vi "HFRR ADV v08.vi"() -> ()   [LabVIEW 2025] (continued)
                  }
                  frame True {
                    w544 = 0.0 ("Major Axis")
                    n250 = Match Pattern(string=w549, regular expression="\"length_px\":") -> (after substring=w547:string)  [unwired: 1 in, 3 out]
                    n251 = property on="Major Axis" class="DigNum (strict)"("Caption.Text"="") -> ()  [unwired: 2 in, 2 out]
                    n252 = property on="Minor Axis" class="DigNum (strict)"("Caption.Text"="") -> ()  [unwired: 2 in, 2 out]
                    n253 = property on="Average" class="DigNum (strict)"("Caption.Text"="Line") -> ()  [unwired: 2 in, 2 out]
                    n254 = Fract/Exp String To Number(string=w547, default (0 dbl)=0.0 ("default (0 DBL)")) -> (number=w543:dbl)  [unwired: 2 in, 1 out]
                    "Pixel Value" <- w543
                    n255 = Multiply(x=w543, y=w545) -> (x*y=w556:dbl)
                    n256 = Multiply(x=w556, y=1000.0) -> (x*y=w539:dbl)
                    n257 = Divide(x=w539, y=1000.0) -> (x/y=w542:dbl)
                    n258 = local write "Measurment (mm)"(w542) -> ()
                    n259 = Bundle By Name(cluster=w548, "average"=w539) -> (w546:cluster{"major":dbl, "minor":dbl, "average":dbl})
                    n260 = Number To Fractional String(number=w539, precision (6)=i16 1) -> (F-format string=w538:string)  [unwired: 2 in]
                    n261 = local write "Minor Axis"(w544) -> ()
                    n262 = local write "Major Axis"(w544) -> ()
                    n263 = Fract/Exp String To Number(string=w538) -> (number=w537:dbl)  [unwired: 3 in, 1 out]
                    n264 = local write "Average"(w537) -> ()
                  }
                }
              }
              frame True {
                w576 = 1000.0 ("y")
                w582 = 0.0 ("default (0 DBL)")
                n265 = Match Pattern(string=w588, regular expression=" \"width_px\":") -> (after substring=w586:string)  [unwired: 1 in, 3 out]
                n266 = Match Pattern(string=w586, regular expression="\"height_px\":") -> (before substring=w584:string, after substring=w583:string)  [unwired: 1 in, 2 out]
                n267 = Fract/Exp String To Number(string=w584, default (0 dbl)=w582) -> (number=w581:dbl)  [unwired: 2 in, 1 out]
                n268 = Fract/Exp String To Number(string=w583, default (0 dbl)=w582) -> (number=w580:dbl)  [unwired: 2 in, 1 out]
                n269 = Multiply(x=w581, y=w579) -> (x*y=w578:dbl)
                n270 = Multiply(x=w580, y=w579) -> (x*y=w577:dbl)
                n271 = Multiply(x=w578, y=w576) -> (x*y=w562:dbl)
                n272 = Multiply(x=w577, y=w576) -> (x*y=w560:dbl)
                n273 = Add(x=w562, y=w560) -> (x+y=w574:dbl)
                n274 = property on="Major Axis" class="DigNum (strict)"("Caption.Text"="Major Axis") -> ()  [unwired: 2 in, 2 out]
                n275 = property on="Minor Axis" class="DigNum (strict)"("Caption.Text"="Minor Axis") -> ()  [unwired: 2 in, 2 out]
                n276 = property on="Average" class="DigNum (strict)"("Caption.Text"="Average") -> ()  [unwired: 2 in, 2 out]
                n277 = Divide(x=w574, y=2.0) -> (x/y=w558:dbl)
                n278 = Bundle By Name(cluster=w575, "major"=w562, "minor"=w560, "average"=w558) -> (w572:cluster{"major":dbl, "minor":dbl, "average":dbl})
                n279 = Number To Fractional String(number=w560, precision (6)=i16 1) -> (F-format string=w567:string)  [unwired: 2 in]
                n280 = Number To Fractional String(number=w558, precision (6)=i16 1) -> (F-format string=w568:string)  [unwired: 2 in]
                n281 = Number To Fractional String(number=w562, precision (6)=i16 1) -> (F-format string=w566:string)  [unwired: 2 in]
                n282 = Fract/Exp String To Number(string=w567) -> (number=w559:dbl)  [unwired: 3 in, 1 out]
                n283 = Fract/Exp String To Number(string=w568) -> (number=w557:dbl)  [unwired: 3 in, 1 out]
                n284 = Fract/Exp String To Number(string=w566) -> (number=w561:dbl)  [unwired: 3 in, 1 out]
                n285 = local write "Major Axis"(w561) -> ()
                n286 = local write "Average"(w557) -> ()
                n287 = local write "Minor Axis"(w559) -> ()
              }
            }
            n288 = case shown="\"Measrument\", Default" w479 {
              tunnel: w482 -> [w506 _]
              tunnel: w481 -> [w505 _]
              tunnel: [w502 w526] -> w480
              tunnel: w478 -> [w504 w526]
              tunnel: w477 -> [w503 _]
              frame "Measrument", Default {
                n289 = stacked-sequence {
                  tunnel: w506 -> [w519 _]
                  tunnel: w505 -> [w517 _]
                  tunnel: w504 -> [w515 _]
                  tunnel: w503 -> [w514 _]
                  tunnel: [w509 _] -> w502
                  frame #0 {
                    n290 = call "IMAGE ANALYSIS.vi"("Enum"=POST_ANALYSIS_ENUM."SAVE IMAGE", "error in"=w515, "IMAGE FILE PATH"=w514) -> ("error out"=w513:errorcluster)  [unwired: 7 in, 1 out]
                    n291 = local read "Test File List :"() -> (w521:string)
                    n292 = call "IMAGE ANALYSIS.vi"("Enum"=POST_ANALYSIS_ENUM."MINIMIZE UI", "error in"=w513) -> ("error out"=w511:errorcluster)  [unwired: 8 in, 1 out]
                    n293 = Bundle By Name(cluster=T18 {"File Name"="", "Test Method"="", "Operator"="", "Fuel Description"="", "Date and time"=""} ("Main Ref"), "File Name"=w521) -> (w522:T18)
                    n294 = call "duf file read.vi"("error in (no error)"=w511, "Main Ref"=w522) -> ("error out"=w520:errorcluster, "Main Ref 2"=w518:T18)  [unwired: 8 in]
                    n295 = call "DETECTION REPORT for manual.vi"("error in (no error)"=w520, "return value 3"=w517, "Image File Path"=w519, "Main Ref"=w518) -> ("error out"=w516:errorcluster)  [unwired: 7 in]
                    n296 = call <vilib>:"Clear Errors.vi"("error in (no error)"=w516) -> ("error out"=w507:errorcluster)  [unwired: 5 in, 1 out]
                    n297 = call "IMAGE ANALYSIS.vi"("Enum"=POST_ANALYSIS_ENUM."MINIMIZE UI", "error in"=w507) -> ("error out"=w509:errorcluster)  [unwired: 8 in, 1 out]
                  }
                  frame #1 {
                    n298 = local write "Main Tab"(T3."HOME" ("Main Tab")) -> ()
                    n299 = local write "Main Dashboard Buttons"(T2."Home" ("Main Dashboard Buttons")) -> ()
                  }
                }
              }
              frame "Calibrate" {
              }
            }
          }
          frame #2 {
            n300 = Not(x=w591) -> (.not. x?=w590:bool)
            n301 = local write "Confirm Measrurement"(w590) -> ()
            n302 = local read "Calibration Tab"() -> (w589:enum32{"Measrument", "Calibrate"})
            n303 = case shown="\"Measrument\", Default" w589 {
              frame "Measrument", Default {
                n304 = local write "Main Tab"(T3."HOME" ("Main Tab")) -> ()
              }
              frame "Calibrate" {
              }
            }
          }
        }
      }
    }
    n305 = local read "Save Change"() -> (w350:bool)
    n306 = local read "Calibrate"() -> (w351:bool)
    n307 = local read "Auto Start Test"() -> (w346:bool)
    n308 = case shown="True" w351 {
      selector: w351 -> [_ w457]
      frame False {
      }
      frame True {
        n309 = Not(x=w457) -> (.not. x?=w456:bool)
        n310 = local write "Calibrate"(w456) -> ()
        n311 = local write "Calibration Tab"(enum32{"Measrument", "Calibrate"}."Calibrate" ("Calibration Tab")) -> ()
      }
    }
    n312 = case shown="True" w350 {
      selector: w350 -> [_ w401]
      frame False {
      }
      frame True {
        n313 = stacked-sequence {
          tunnel: w401 -> [_ _ _ _ w455]
          frame #0 {
            n314 = call "IMAGE ANALYSIS.vi"("Enum"=POST_ANALYSIS_ENUM."HIDE UI") -> ()  [unwired: 9 in, 2 out]
          }
          frame #1 {
            n315 = local read "100x gain"() -> (w403:dbl)
            n316 = local read "10x Gain"() -> (w404:dbl)
            n317 = local read "5x Gain"() -> (w405:dbl)
            n318 = Number To Fractional String(number=w404, width (-)=i16 4, precision (6)=i16 7) -> (F-format string=w426:string)  [unwired: 1 in]
            n319 = Number To Fractional String(number=0.0, width (-)=i16 4, precision (6)=i16 7) -> (F-format string=w421:string)  [unwired: 1 in]
            n320 = Number To Fractional String(number=w403, width (-)=i16 4, precision (6)=i16 7) -> (F-format string=w409:string)  [unwired: 1 in]
            n321 = Number To Fractional String(number=w405, width (-)=i16 10 ("precision (6)"), precision (6)=i16 7) -> (F-format string=w435:string)  [unwired: 1 in]
            n322 = Concatenate Strings("[CH1]" ("string"), w435, " - 5x Gain" ("string"), "\r") -> (w425:string)
            n323 = Concatenate Strings("[CH2]" ("string"), w426, " - 10x Gain" ("string"), "\r") -> (w424:string)
            n324 = Concatenate Strings("[CH3]" ("string"), w421, " - 20x Gain" ("string"), "\r") -> (w415:string)
            n325 = Concatenate Strings("[CH4]" ("string"), w409, " - 100x Gain" ("string"), "\r") -> (w408:string)
            n326 = String To Path(string="C:\\LAB-IQ\\Image Calibrate v01.dcf") -> (path=w438:path)
            n327 = Concatenate Strings(w425, w424, w415, w408) -> (w423:string)
            n328 = call <vilib>:"Write Characters To File.vi"("append to file? (new file:F)"=FALSE, "character string"=w423, "file path (dialog if empty)"=w438) -> ()  [unwired: 2 in, 1 out]
          }
          frame #2 {
            n329 = String To Path(string="C:\\LAB-IQ\\Image Calibrate v01.dcf") -> (path=w441:path)
            n330 = Open/Create/Replace File ("Open File")(file path (use dialog)=w441) -> (refnum out=w442:refnum<file>)  [unwired: 5 in, 2 out]
            n331 = for {
              N: 4 -> [_]
              tunnel: w442 -> [w448]
              i -> [w444]
              n332 = Read from Text File ("Read File")(file (use dialog)=w448) -> (text=w449:string)  [unwired: 3 in, 3 out]
              n333 = String Subset(string=w449, offset (0)=6, length (rest)=10 ("length (rest)")) -> (substring=w445:string)
              n334 = Fract/Exp String To Number(string=w445) -> (number=w443:dbl)  [unwired: 3 in, 1 out]
              n335 = case shown="3" w444 {
                tunnel: w443 -> [w450 w451 _ w452 _]
                frame 0 {
                  n336 = local write "5x Gain"(w450) -> ()
                }
                frame 1 {
                  n337 = local write "10x Gain"(w451) -> ()
                }
                frame 2 {
                }
                frame 3 {
                  n338 = local write "100x gain"(w452) -> ()
                }
                frame 4, Default {
                }
              }
            }
          }
          frame #3 {
            n339 = call "IMAGE ANALYSIS.vi"("Enum"=POST_ANALYSIS_ENUM."SHOW UI") -> ()  [unwired: 9 in, 2 out]
          }
          frame #4 {
            n340 = Not(x=w455) -> (.not. x?=w454:bool)
            n341 = local write "Save Change"(w454) -> ()
          }
        }
      }
    }
    n342 = case shown="True" w346 {
      frame False {
        n343 = local read "Set Humidity:"() -> (w375:dbl)
        n344 = local read "Set Humidity:"() -> (w378:dbl)
        n345 = local read "Humidity ( %RH )"() -> (w379:dbl)
        n346 = Subtract(x=w375, y=1.0) -> (x-y=w373:dbl)
        n347 = Add(x=w378, y=1.0) -> (x+y=w374:dbl)
        n348 = In Range and Coerce(upper limit=w374, x=w379, lower limit=w373) -> (In Range?=w372:bool)  [unwired: 1 out]
        n349 = case shown="True" w372 {
          frame False {
          }
          frame True {
            n350 = case shown="True" "Manual Humididty Reached" {
              selector: "Manual Humididty Reached" -> [_ w382]
              frame False {
              }
              frame True {
                n351 = Not(x=w382) -> (.not. x?=w381:bool)
                n352 = local write "Manual Humididty Reached"(w381) -> ()
                n353 = local read "EVENT LOG"() -> (w384:string)
                n354 = call "Event Log.vi"("Content"="Target Humidity reached", "EVENT LOG"=w384) -> ("EVENT LOG"=w383:string)  [unwired: 8 in, 1 out]
                n355 = local write "EVENT LOG"(w383) -> ()
              }
            }
          }
        }
      }
      frame True {
        n356 = local write "Manual Humididty Reached"(TRUE ("Manual Humididty Reached")) -> ()
      }
    }
    n357 = local read "Cap Live Image"() -> (w366:bool)
    n358 = local read "SCAR MEASURMENT"() -> (w369:enum32{"Auto Scar", "Manual Scar"})
    n359 = Wait (ms)(milliseconds to wait=u32 250) -> ()  [unwired: 1 out]
    n360 = Equal?(x=w369, y=enum32{"Auto Scar", "Manual Scar"}."Manual Scar" ("SCAR MEASURMENT")) -> (x = y?=w367:bool)
    n361 = And(x=w367, y=w366) -> (x .and. y?=w365:bool)
    n362 = case shown="True" w365 {
      selector: w365 -> [_ w670]
      frame False {
      }
      frame True {
        n363 = stacked-sequence {
          tunnel: [_ _ _ w685 _] -> _
          tunnel: w670 -> [_ _ _ _ w691]
          frame #0 {
            w671 = 0.0
            n364 = local write "Major Axis"(w671) -> ()
            n365 = local write "Minor Axis"(w671) -> ()
            n366 = local write "Average"(w671) -> ()
          }
          frame #1 {
            n367 = call "CAMERA LIVE FEED FGV.vi"("Enum - Menu"=CAMERA_LIVE_FEED_ENUM."CAMERA MINIMIZE") -> ()  [unwired: 9 in, 2 out]
          }
          frame #2 {
            n368 = local read "FILE 3"() -> (w679:string)
            n369 = call <vilib>:"Trim Whitespace.vi"("string"="C:\\LAB-IQ\\images\\") -> ("trimmed string"=w681:string)  [unwired: 1 in]
            n370 = String To Path(string=w681) -> (path=w680:path)
            n371 = Concatenate Strings(w679, ".png" ("string")) -> (w678:string)
            n372 = Build Path(base path=w680, name or relative path=w678) -> (appended path=w676:path)
            n373 = Path To String(path=w676) -> (string=w675:string)
            n374 = call "CAMERA LIVE FEED FGV.vi"("Enum - Menu"=CAMERA_LIVE_FEED_ENUM."CAMERA SAVE", "Image Path"=w675) -> ("error out"=w673:errorcluster)  [unwired: 8 in, 1 out]
            n375 = case shown="No Error" w673 {
              frame No Error {
                n376 = One Button Dialog(message="Image saved successfully") -> ()  [unwired: 1 in, 1 out]
              }
              frame Error {
              }
            }
          }
          frame #3 {
            n377 = call "LIST FILE NAMES.vi"() -> ("error out"=w687:errorcluster, "filenames"=w684:string[])  [unwired: 10 in]
            n378 = call "IMAGE ANALYSIS.vi"("Enum"=POST_ANALYSIS_ENUM."SHOW UI", "error in"=w687) -> ("error out"=w685:errorcluster)  [unwired: 8 in, 1 out]
            n379 = property on="Test File List :" class="CmbBox"("Strings[]"=w684) -> ()  [unwired: 2 in, 2 out]
          }
          frame #4 {
            n380 = Not(x=w691) -> (.not. x?=w690:bool)
            n381 = local write "Zoom Factore"(0.0 ("Zoom Factore")) -> ()
            n382 = local write "Cap Live Image"(w690) -> ()
            n383 = local write "Main Tab"(T3."Adv Scar Report" ("Main Tab")) -> ()
            n384 = local write "Main Dashboard Buttons"(T2."Report" ("Main Dashboard Buttons")) -> ()
            n385 = property on="Cap Live Image" class="Bool (strict)"("BoolText.Text"="Capture Image" ("Boolean Text.Text")) -> ()  [unwired: 2 in, 2 out]
          }
        }
      }
    }
    n386 = local read "change Gain"() -> (w349:bool)
    n387 = local read "Back Square"() -> (w348:bool)
    n388 = case shown="True" w349 {
      selector: w349 -> [_ w392]
      frame False {
      }
      frame True {
        n389 = stacked-sequence {
          tunnel: w392 -> [_ w400]
          frame #0 {
            n390 = local read "Actual (µm)"() -> (w396:dbl)
            n391 = local read "Pixel Value"() -> (w395:dbl)
            n392 = local read "Magnification :"() -> (w394:string)
            n393 = Divide(x=w396, y=w395) -> (x/y=w393:dbl)
            n394 = case shown="\"10x\"" w394 {
              tunnel: w393 -> [w397 w398]
              frame "10x" {
                n395 = local write "10x Gain"(w397) -> ()
              }
              frame "5x", Default {
                n396 = local write "5x Gain"(w398) -> ()
              }
            }
          }
          frame #1 {
            n397 = Not(x=w400) -> (.not. x?=w399:bool)
            n398 = local write "change Gain"(w399) -> ()
          }
        }
      }
    }
    n399 = case shown="True" w348 {
      selector: w348 -> [_ w390]
      frame False {
      }
      frame True {
        n400 = Not(x=w390) -> (.not. x?=w389:bool)
        n401 = local write "Back Square"(w389) -> ()
        n402 = local write "Calibration Tab"(enum32{"Measrument", "Calibrate"}."Measrument" ("Calibration Tab")) -> ()
      }
    }
    n403 = local read "Rectangle Tool"() -> (w360:bool)
    n404 = local read "Clear ROI Tool"() -> (w359:bool)
    n405 = local read "Open Image"() -> (w364:bool)
    n406 = local read "line tool"() -> (w361:bool)
    n407 = local read "OUT"() -> (w362:bool)
    n408 = local read "In"() -> (w363:bool)
    n409 = case shown="True" w364 {
      selector: w364 -> [_ w658]
      tunnel: [w654 w660] -> _
      tunnel: w354 -> [w654 w659]
      frame False {
      }
      frame True {
        n410 = Not(x=w658) -> (.not. x?=w657:bool)
        n411 = local write "Open Image"(w657) -> ()
        n412 = call "IMAGE ANALYSIS.vi"("Enum"=POST_ANALYSIS_ENUM."HIDE UI", "error in"=w659) -> ("error out"=w667:errorcluster)  [unwired: 8 in, 1 out]
        n413 = call "File Dialog"("start path"=path "C:/LAB-IQ/images", "error in"=w667) -> ("selected path"=w656:path, "error out"=w665:errorcluster)  [unwired: 10 in, 2 out]
        "Image path" <- w656
        n414 = call <vilib>:"Clear Errors.vi"("error in (no error)"=w665) -> ("error out"=w664:errorcluster)  [unwired: 5 in, 1 out]
        n415 = call "IMAGE ANALYSIS.vi"("Enum"=POST_ANALYSIS_ENUM."OPEN FILE", "error in"=w664, "File Path"=w656) -> ("error out"=w663:errorcluster)  [unwired: 7 in, 1 out]
        n416 = call <vilib>:"Clear Errors.vi"("error in (no error)"=w663) -> ("error out"=w662:errorcluster)  [unwired: 5 in, 1 out]
        n417 = call "IMAGE ANALYSIS.vi"("Enum"=POST_ANALYSIS_ENUM."SHOW UI", "error in"=w662) -> ("error out"=w660:errorcluster)  [unwired: 8 in, 1 out]
        n418 = local write "Zoom Factore"(100.0 ("Zoom Factore")) -> ()
      }
    }
    n419 = case shown="True" w362 {
      selector: w362 -> [_ w639]
      tunnel: w354 -> [w636 w644]
      tunnel: [w636 w638] -> _
      frame False {
      }
      frame True {
        n420 = Not(x=w639) -> (.not. x?=w637:bool)
        n421 = local read "Zoom Factore"() -> (w642:dbl)
        n422 = local write "OUT"(w637) -> ()
        n423 = call "IMAGE ANALYSIS.vi"("Enum"=POST_ANALYSIS_ENUM."ZOOM OUT", "error in"=w644) -> ("error out"=w638:errorcluster)  [unwired: 8 in, 1 out]
        n424 = Divide(x=w642, y=1.2) -> (x/y=w640:dbl)
        n425 = local write "Zoom Factore"(w640) -> ()
      }
    }
    n426 = case shown="True" w363 {
      selector: w363 -> [_ w648]
      tunnel: w354 -> [w645 w653]
      tunnel: [w645 w646] -> _
      frame False {
      }
      frame True {
        n427 = Not(x=w648) -> (.not. x?=w647:bool)
        n428 = local read "Zoom Factore"() -> (w651:dbl)
        n429 = local write "In"(w647) -> ()
        n430 = call "IMAGE ANALYSIS.vi"("Enum"=POST_ANALYSIS_ENUM."ZOOM IN", "error in"=w653) -> ("error out"=w646:errorcluster)  [unwired: 8 in, 1 out]
        n431 = Multiply(x=w651, y=1.2) -> (x*y=w649:dbl)
        n432 = local write "Zoom Factore"(w649) -> ()
      }
    }
    n433 = case shown="True" w359 {
      selector: w359 -> [_ w620]
      tunnel: w354 -> [w618 w622]
      tunnel: [w618 w621] -> _
      frame False {
      }
      frame True {
        n434 = Not(x=w620) -> (.not. x?=w619:bool)
        n435 = local write "Clear ROI Tool"(w619) -> ()
        n436 = call "IMAGE ANALYSIS.vi"("Enum"=POST_ANALYSIS_ENUM."CLEAR ROI", "error in"=w622) -> ("error out"=w621:errorcluster)  [unwired: 8 in, 1 out]
      }
    }
    n437 = case shown="True" w361 {
      selector: w361 -> [_ w632]
      tunnel: w354 -> [w630 w635]
      tunnel: [w630 w633] -> _
      frame False {
      }
      frame True {
        n438 = Not(x=w632) -> (.not. x?=w631:bool)
        n439 = local write "line tool"(w631) -> ()
        n440 = call "IMAGE ANALYSIS.vi"("Enum"=POST_ANALYSIS_ENUM."DRAW LINE", "error in"=w635) -> ("error out"=w633:errorcluster)  [unwired: 8 in, 1 out]
      }
    }
    n441 = case shown="True" w360 {
      selector: w360 -> [_ w626]
      tunnel: w354 -> [w624 w628]
      tunnel: [w624 w627] -> _
      frame False {
      }
      frame True {
        n442 = Not(x=w626) -> (.not. x?=w625:bool)
        n443 = local write "Rectangle Tool"(w625) -> ()
        n444 = call "IMAGE ANALYSIS.vi"("Enum"=POST_ANALYSIS_ENUM."DRAW REC", "error in"=w628) -> ("error out"=w627:errorcluster)  [unwired: 8 in, 1 out]
      }
    }
    n445 = local read "SCAR MEASURMENT"() -> (w347:enum32{"Auto Scar", "Manual Scar"})
    n446 = local read "Fit to Screen Tool"() -> (w356:bool)
    n447 = local read "Resize Tool"() -> (w355:bool)
    n448 = case shown="\"Manual Scar\"" w347 {
      frame "Auto Scar", Default {
        n449 = property on="Cap Live Image" class="Bool (strict)"("BoolText.Text"="Report" ("Boolean Text.Text")) -> ()  [unwired: 2 in, 2 out]
      }
      frame "Manual Scar" {
        n450 = property on="Cap Live Image" class="Bool (strict)"("BoolText.Text"="Save Image" ("Boolean Text.Text")) -> ()  [unwired: 2 in, 2 out]
      }
    }
    n451 = local read "ROI Color Tool"() -> (w357:bool)
    n452 = local read "Pan Tool"() -> (w358:bool)
    n453 = case shown="True" w358 {
      selector: w358 -> [_ w614]
      tunnel: w354 -> [w612 w616]
      tunnel: [w612 w615] -> _
      frame False {
      }
      frame True {
        n454 = Not(x=w614) -> (.not. x?=w613:bool)
        n455 = call "IMAGE ANALYSIS.vi"("Enum"=POST_ANALYSIS_ENUM."PAN", "error in"=w616) -> ("error out"=w615:errorcluster)  [unwired: 8 in, 1 out]
        n456 = local write "Pan Tool"(w613) -> ()
      }
    }
    n457 = case shown="True" w355 {
      selector: w355 -> [_ w598]
      tunnel: w354 -> [w593 w595]
      tunnel: [w593 w594] -> _
      frame False {
      }
      frame True {
        n458 = Not(x=w598) -> (.not. x?=w597:bool)
        n459 = local write "Resize Tool"(w597) -> ()
        n460 = call "IMAGE ANALYSIS.vi"("Enum"=POST_ANALYSIS_ENUM."RESIZE MODE", "error in"=w595) -> ("error out"=w594:errorcluster)  [unwired: 8 in, 1 out]
      }
    }
    n461 = case shown="True" w356 {
      selector: w356 -> [_ w603]
      tunnel: [w599 w604] -> _
      tunnel: w354 -> [w599 w602]
      frame False {
      }
      frame True {
        n462 = Not(x=w603) -> (.not. x?=w601:bool)
        n463 = local write "Zoom Factore"(100.0 ("Zoom Factore")) -> ()
        n464 = local write "Fit to Screen Tool"(w601) -> ()
        n465 = call "IMAGE ANALYSIS.vi"("Enum"=POST_ANALYSIS_ENUM."FIT", "error in"=w602) -> ("error out"=w604:errorcluster)  [unwired: 8 in, 1 out]
      }
    }
    n466 = case shown="True" w357 {
      selector: w357 -> [_ w609]
      tunnel: [w606 w610] -> _
      tunnel: w354 -> [w606 w607]
      frame False {
      }
      frame True {
        n467 = Not(x=w609) -> (.not. x?=w608:bool)
        n468 = local write "ROI Color Tool"(w608) -> ()
        n469 = call "IMAGE ANALYSIS.vi"("Enum"=POST_ANALYSIS_ENUM."SET ROI COLOR", "error in"=w607) -> ("error out"=w610:errorcluster)  [unwired: 8 in, 1 out]
      }
    }
    n470 = local read "Quit"() -> (w371:bool)
  }
  n471 = while {
    stop <- w694 stop-if-true
    n472 = event shown="[3] \"Auto Start Test\": Value Change" {
      selector: _ -> [_ _ _ _ _]
      dyn-events: _ -> [_ _ _ _ _]
      timeout: 100 -> [_ _ _ _ _]
      tunnel: [FALSE FALSE _ FALSE TRUE] -> w694
      event Timeout {
        n473 = event-data() -> ()  [unwired: 1 in, 3 out]
        n474 = Get Date/Time In Seconds() -> (seconds since 1Jan1904=w699:timestamp)
        n475 = Format Into String(format string="%<%I:%M:%S:%p %d:%B:%Y>T", w699) -> (resulting string=→"Time Stamp":string)  [unwired: 2 in, 1 out]
      }
      event "RUN": Value Change {
        n476 = event-data() -> ()  [unwired: 1 in, 6 out]
        n477 = local read "RUN"() -> (w702:bool)
        n478 = case shown="False" w702 {
          frame False {
            n479 = property on="Auto Start Test" class="Bool (strict)"("Visible"=TRUE) -> ()  [unwired: 2 in, 2 out]
          }
          frame True {
            n480 = property on="Auto Start Test" class="Bool (strict)"("Visible"=FALSE) -> ()  [unwired: 2 in, 2 out]
          }
        }
      }
      event "Auto": Value Change {
        n481 = event-data() -> ()  [unwired: 1 in, 6 out]
        n482 = stacked-sequence {
          frame #0 {
            n483 = local write "FILE"("") -> ()
          }
          frame #1 {
            n484 = Get Date/Time In Seconds() -> (seconds since 1Jan1904=w709:timestamp)
            n485 = Format Into String(format string="%<%I_%M_%S_%p_%d_%B_%Y>T", w709) -> (resulting string=w708:string)  [unwired: 2 in, 1 out]
            n486 = local write "FILE"(w708) -> ()
          }
        }
        n487 = local read "Auto"() -> (w706:bool)
        n488 = Not(x=w706) -> (.not. x?=w705:bool)
        n489 = local write "Auto"(w705) -> ()
      }
      event "Auto Start Test": Value Change {
        n490 = event-data() -> ()  [unwired: 1 in, 6 out]
        n491 = local read "Auto Start Test"() -> (w712:bool)
        n492 = case shown="False" w712 {
          frame False {
            n493 = property on="RUN" class="Bool (strict)"("Visible"=TRUE) -> ()  [unwired: 2 in, 2 out]
          }
          frame True {
            n494 = property on="RUN" class="Bool (strict)"("Visible"=FALSE) -> ()  [unwired: 2 in, 2 out]
          }
        }
      }
      event "Quit": Value Change {
        n495 = event-data() -> ()  [unwired: 1 in, 6 out]
      }
    }
    n496 = Wait (ms)(milliseconds to wait=u32 100) -> ()  [unwired: 1 out]
  }
  n497 = local write "Temperature Off Command"(w6) -> ()
  n498 = local write "Main Dashboard Buttons"(T2."Home" ("Main Dashboard Buttons")) -> ()
  n499 = local write "Humidity Off Command"(w6) -> ()
  n500 = local write "CAMERA ROI MIN TEMP"(w6) -> ()
  n501 = local write "LIVE FEED MIN TEMP"(w6) -> ()
  n502 = local write "Auto stop temp"(w2) -> ()
  n503 = local write "main tab sub"(enum32{"Page 1", "Page 2"}."Page 1" ("main tab sub")) -> ()
  n504 = local write "USERNAME"(w21) -> ()
  n505 = local write "Main Tab"(T3."HOME" ("Main Tab")) -> ()
  n506 = local write "USER ID"(w21) -> ()
  n507 = property on="Auto Scar Check  2" class="Clust (strict)"("Visible"=w2) -> (error out=w4:errorcluster)  [unwired: 2 in, 1 out]
  n508 = property on="Quit" class="Bool (strict)"("Value"=FALSE ("Quit")) -> (error out=w23:errorcluster)  [unwired: 2 in, 1 out]
  n509 = while {
    stop <- w716 stop-if-true
    n510 = local read "Image Path"() -> (w719:path)
    n511 = local read "Print 3"() -> (w722:bool)
    n512 = Equal?(x=w719, y=path "") -> (x = y?=w718:bool)
    n513 = Not(x=w718) -> (.not. x?=w717:bool)
    n514 = property on="Print 3" class="Bool (strict)"("Visible"=w717) -> ()  [unwired: 2 in, 2 out]
    n515 = case shown="True" w722 {
      frame False {
        n516 = local write "Rd"(TRUE ("Boolean 7")) -> ()
      }
      frame True {
        n517 = flat-sequence {
          tunnel: [w762] -> w730
          tunnel: [w749] -> w728
          tunnel: [w759] -> w724
          tunnel: w730 -> [w771]
          tunnel: [w771] -> w729
          tunnel: w728 -> [w770]
          tunnel: [w770] -> w727
          tunnel: [w768] -> w726
          tunnel: [w767] -> w725
          tunnel: w724 -> [w767]
          tunnel: w729 -> [w773]
          tunnel: w727 -> [w774]
          tunnel: w726 -> [_]
          tunnel: w725 -> [w772]
          frame #0 {
            n518 = case shown="True" "Rd" {
              frame False {
              }
              frame True {
                n519 = while {
                  tunnel: "abcdefABCDEF" ("string 2") -> [w741]
                  shift-right: [w739] -> w733
                  shift-left: "" -> [w738]
                  i -> [w748]
                  stop <- w747 stop-if-true
                  n520 = Random Number (0-1)() -> (number: 0 to 1=w742:dbl)
                  n521 = Multiply(x=w742, y=62.0) -> (x*y=w744:dbl)
                  n522 = Decrement(x="Length 2") -> (x-1=w737:i16)
                  n523 = To Word Integer(number=w744) -> (16bit integer=w745:i16)
                  n524 = String Subset(string=w741, offset (0)=w745, length (rest)=1 ("length (rest)")) -> (substring=w740:string)
                  n525 = Greater Or Equal?(x=w748, y=w737) -> (x >= y?=w747:bool)
                  n526 = Concatenate Strings(w740, w738) -> (w739:string)
                }
                "String 10" <- w733
                n527 = local write "Rd"(FALSE ("Boolean 7")) -> ()
              }
            }
          }
          frame #1 {
            w760 = "_resized.jpg" ("command line")
            (unwired) ".jpg -resize 320x240 " ("string")
            (unwired) "Choose an Image File" ("prompt")
            # "-resize 1798x425"
            n528 = local read "Image Path"() -> (w754:path)
            n529 = Strip Path(path=w754) -> (stripped path=w749:path, name=w750:string)
            n530 = Match Pattern(string=w750, regular expression=".jpg") -> (before substring=→"before substring 2":string, after substring=→"after substring":string)  [unwired: 1 in, 2 out]
            n531 = Match Pattern(string=w750, regular expression="\\") -> (before substring=w756:string)  [unwired: 1 in, 3 out]
            n532 = Match Pattern(string=w756, regular expression=".jpg") -> (before substring=w755:string)  [unwired: 1 in, 3 out]
            n533 = Concatenate Strings("cmd /c convert " ("string"), w755, ".jpg -resize 320x240  " ("command line"), w755, w760) -> (w763:string)
            n534 = call <vilib>:"System Exec.vi"("run minimized? (F)"=TRUE, "wait until completion? (T)"=TRUE, "working directory"=w749, "command line"=w763) -> ("error out"=w762:errorcluster)  [unwired: 4 in, 3 out]
            "error out 2" <- w762
            n535 = Concatenate Strings(w755, w760) -> (w759:string)
          }
          frame #2 {
            n536 = Wait (ms)(milliseconds to wait=u32 2000 ("millisecond timer value")) -> (millisecond timer value=w768:u32)
          }
          frame #3 {
            n537 = case shown="No Error" w773 {
              tunnel: w774 -> [w777 _]
              tunnel: w772 -> [w775 _]
              frame No Error {
                (unwired) ".jpg" ("string")
                n538 = Path To String(path=w777) -> (string=w781:string)
                n539 = Concatenate Strings(w781, "\\" ("string"), w775) -> (w780:string)
                n540 = String To Path(string=w780) -> (path=w779:path)
                n541 = call <vilib>:"Read JPEG File.vi"("path to JPEG file"=w779) -> ("image data"=w783:T12)  [unwired: 8 in, 2 out]
                "image data" <- w783
                n542 = local write "Print 3"(FALSE ("Print 2")) -> ()
                n543 = call <vilib>:"Draw Flattened Pixmap.vi"("image data"=w783) -> ("new picture"=→"new picture":picture)  [unwired: 8 in]
              }
              frame Error {
              }
            }
          }
        }
      }
    }
    n544 = Wait (ms)(milliseconds to wait=u32 20 ("millisecond timer value")) -> ()  [unwired: 1 out]
    n545 = local read "Quit"() -> (w716:bool)
  }
  n546 = while {
    tunnel: w23 -> [_]
    tunnel: w4 -> [_]
    stop <- w814 stop-if-true
    # "New Adv Logics"
    n547 = local read "Main Tab"() -> (w812:T3)
    n548 = local read "Sign In"() -> (w811:bool)
    n549 = local read "Main Tab"() -> (w793:T3)
    n550 = case shown="\"About\"" w793 {
      frame "HOME", Default {
        n551 = local read "LIVE FEED MIN TEMP"() -> (w888:bool)
        n552 = local write "LIVE FEED MAX TEMP"(TRUE ("LIVE FEED MAX TEMP")) -> ()
        n553 = local read "CAMERA ROI MIN TEMP"() -> (w886:bool)
        n554 = case shown="True" w888 {
          selector: w888 -> [_ w895]
          frame False {
          }
          frame True {
            n555 = Not(x=w895) -> (.not. x?=w894:bool)
            n556 = local write "LIVE FEED MIN TEMP"(w894) -> ()
            n557 = call "CAMERA LIVE FEED FGV.vi"("Enum - Menu"=CAMERA_LIVE_FEED_ENUM."CAMERA MINIMIZE") -> ()  [unwired: 9 in, 2 out]
          }
        }
        n558 = case shown="True" w886 {
          selector: w886 -> [_ w892]
          frame False {
          }
          frame True {
            n559 = Not(x=w892) -> (.not. x?=w891:bool)
            n560 = local write "CAMERA ROI MIN TEMP"(w891) -> ()
            n561 = call "IMAGE ANALYSIS.vi"("Enum"=POST_ANALYSIS_ENUM."MINIMIZE UI") -> ()  [unwired: 9 in, 2 out]
          }
        }
        n562 = local write "CAMERA ROI MAX TEMP"(TRUE ("CAMERA ROI MAX TEMP")) -> ()
      }
      frame "Test Setup" {
        n563 = local read "LIVE FEED MIN TEMP"() -> (w898:bool)
        n564 = local read "CAMERA ROI MIN TEMP"() -> (w896:bool)
        n565 = local write "LIVE FEED MAX TEMP"(TRUE ("LIVE FEED MAX TEMP")) -> ()
        n566 = case shown="True" w898 {
          selector: w898 -> [_ w905]
          frame False {
          }
          frame True {
            n567 = Not(x=w905) -> (.not. x?=w904:bool)
            n568 = local write "LIVE FEED MIN TEMP"(w904) -> ()
            n569 = call "CAMERA LIVE FEED FGV.vi"("Enum - Menu"=CAMERA_LIVE_FEED_ENUM."CAMERA MINIMIZE") -> ()  [unwired: 9 in, 2 out]
          }
        }
        n570 = case shown="True" w896 {
          selector: w896 -> [_ w902]
          frame False {
          }
          frame True {
            n571 = Not(x=w902) -> (.not. x?=w901:bool)
            n572 = local write "CAMERA ROI MIN TEMP"(w901) -> ()
            n573 = call "IMAGE ANALYSIS.vi"("Enum"=POST_ANALYSIS_ENUM."MINIMIZE UI") -> ()  [unwired: 9 in, 2 out]
          }
        }
        n574 = local write "CAMERA ROI MAX TEMP"(TRUE ("CAMERA ROI MAX TEMP")) -> ()
      }
      frame "Acquire" {
        n575 = local read "LIVE FEED MIN TEMP"() -> (w908:bool)
        n576 = local write "LIVE FEED MAX TEMP"(TRUE ("LIVE FEED MAX TEMP")) -> ()
        n577 = local read "CAMERA ROI MIN TEMP"() -> (w906:bool)
        n578 = case shown="True" w908 {
          selector: w908 -> [_ w915]
          frame False {
          }
          frame True {
            n579 = Not(x=w915) -> (.not. x?=w914:bool)
            n580 = local write "LIVE FEED MIN TEMP"(w914) -> ()
            n581 = call "CAMERA LIVE FEED FGV.vi"("Enum - Menu"=CAMERA_LIVE_FEED_ENUM."CAMERA MINIMIZE") -> ()  [unwired: 9 in, 2 out]
          }
        }
        n582 = case shown="True" w906 {
          selector: w906 -> [_ w912]
          frame False {
          }
          frame True {
            n583 = Not(x=w912) -> (.not. x?=w911:bool)
            n584 = local write "CAMERA ROI MIN TEMP"(w911) -> ()
            n585 = call "IMAGE ANALYSIS.vi"("Enum"=POST_ANALYSIS_ENUM."MINIMIZE UI") -> ()  [unwired: 9 in, 2 out]
          }
        }
        n586 = local write "CAMERA ROI MAX TEMP"(TRUE ("CAMERA ROI MAX TEMP")) -> ()
      }
      frame "Adv Scar" {
        n587 = local read "CAMERA ROI MIN TEMP"() -> (w916:bool)
        n588 = case shown="True" "LIVE FEED MAX TEMP" {
          selector: "LIVE FEED MAX TEMP" -> [_ w928]
          frame False {
          }
          frame True {
            n589 = Not(x=w928) -> (.not. x?=w927:bool)
            n590 = local write "LIVE FEED MAX TEMP"(w927) -> ()
            n591 = call "CAMERA LIVE FEED FGV.vi"("Enum - Menu"=CAMERA_LIVE_FEED_ENUM."CAMERA RESTORE") -> ("error out"=w923:errorcluster)  [unwired: 9 in, 1 out]
            n592 = call "LIST FILE NAMES.vi"("error in (no error)"=w923) -> ("error out"=w924:errorcluster, "filenames"=w925:string[])  [unwired: 9 in]
            n593 = property on="FILE 3" class="CmbBox"(error in=w924, "Strings[]"=w925) -> ()  [unwired: 1 in, 2 out]
          }
        }
        n594 = case shown="True" w916 {
          selector: w916 -> [_ w922]
          frame False {
          }
          frame True {
            n595 = Not(x=w922) -> (.not. x?=w921:bool)
            n596 = local write "CAMERA ROI MIN TEMP"(w921) -> ()
            n597 = call "IMAGE ANALYSIS.vi"("Enum"=POST_ANALYSIS_ENUM."MINIMIZE UI") -> ()  [unwired: 9 in, 2 out]
          }
        }
        n598 = local write "CAMERA ROI MAX TEMP"(TRUE ("CAMERA ROI MAX TEMP")) -> ()
        "LIVE FEED MIN TEMP" <- TRUE ("LIVE FEED MIN TEMP")
      }
      frame "Adv Scar Report" {
        n599 = local read "CAMERA ROI MAX TEMP"() -> (w929:bool)
        n600 = local read "LIVE FEED MIN TEMP"() -> (w931:bool)
        n601 = local write "LIVE FEED MAX TEMP"(TRUE ("LIVE FEED MAX TEMP")) -> ()
        n602 = case shown="True" w931 {
          selector: w931 -> [_ w940]
          frame False {
          }
          frame True {
            n603 = Not(x=w940) -> (.not. x?=w939:bool)
            n604 = local write "LIVE FEED MIN TEMP"(w939) -> ()
            n605 = call "CAMERA LIVE FEED FGV.vi"("Enum - Menu"=CAMERA_LIVE_FEED_ENUM."CAMERA MINIMIZE") -> ()  [unwired: 9 in, 2 out]
          }
        }
        n606 = case shown="True" w929 {
          selector: w929 -> [_ w937]
          frame False {
          }
          frame True {
            n607 = Not(x=w937) -> (.not. x?=w935:bool)
            n608 = local write "CAMERA ROI MAX TEMP"(w935) -> ()
            n609 = call "IMAGE ANALYSIS.vi"("Enum"=POST_ANALYSIS_ENUM."SHOW UI") -> ("error out"=w934:errorcluster)  [unwired: 9 in, 1 out]
            n610 = call "LIST FILE NAMES.vi"("error in (no error)"=w934) -> ("filenames"=w933:string[])  [unwired: 9 in, 1 out]
            n611 = property on="Test File List :" class="CmbBox"("Strings[]"=w933) -> ()  [unwired: 2 in, 2 out]
          }
        }
        n612 = local write "CAMERA ROI MIN TEMP"(TRUE ("CAMERA ROI MIN TEMP")) -> ()
      }
      frame "Compare Files" {
        n613 = local read "LIVE FEED MIN TEMP"() -> (w943:bool)
        n614 = local write "LIVE FEED MAX TEMP"(TRUE ("LIVE FEED MAX TEMP")) -> ()
        n615 = local read "CAMERA ROI MIN TEMP"() -> (w941:bool)
        n616 = case shown="True" w943 {
          selector: w943 -> [_ w950]
          frame False {
          }
          frame True {
            n617 = Not(x=w950) -> (.not. x?=w949:bool)
            n618 = local write "LIVE FEED MIN TEMP"(w949) -> ()
            n619 = call "CAMERA LIVE FEED FGV.vi"("Enum - Menu"=CAMERA_LIVE_FEED_ENUM."CAMERA MINIMIZE") -> ()  [unwired: 9 in, 2 out]
          }
        }
        n620 = case shown="True" w941 {
          selector: w941 -> [_ w947]
          frame False {
          }
          frame True {
            n621 = Not(x=w947) -> (.not. x?=w946:bool)
            n622 = local write "CAMERA ROI MIN TEMP"(w946) -> ()
            n623 = call "IMAGE ANALYSIS.vi"("Enum"=POST_ANALYSIS_ENUM."MINIMIZE UI") -> ()  [unwired: 9 in, 2 out]
          }
        }
        n624 = local write "CAMERA ROI MAX TEMP"(TRUE ("CAMERA ROI MAX TEMP")) -> ()
      }
      frame "About" {
        n625 = local read "LIVE FEED MIN TEMP"() -> (w953:bool)
        n626 = local write "LIVE FEED MAX TEMP"(TRUE ("LIVE FEED MAX TEMP")) -> ()
        n627 = local read "CAMERA ROI MIN TEMP"() -> (w952:bool)
        n628 = case shown="True" w953 {
          selector: w953 -> [_ w960]
          frame False {
          }
          frame True {
            n629 = Not(x=w960) -> (.not. x?=w959:bool)
            n630 = local write "LIVE FEED MIN TEMP"(w959) -> ()
            n631 = call "CAMERA LIVE FEED FGV.vi"("Enum - Menu"=CAMERA_LIVE_FEED_ENUM."CAMERA MINIMIZE") -> ()  [unwired: 9 in, 2 out]
          }
        }
        n632 = case shown="True" w952 {
          selector: w952 -> [_ w957]
          frame False {
          }
          frame True {
            n633 = Not(x=w957) -> (.not. x?=w956:bool)
            n634 = local write "CAMERA ROI MIN TEMP"(w956) -> ()
            n635 = call "IMAGE ANALYSIS.vi"("Enum"=POST_ANALYSIS_ENUM."MINIMIZE UI") -> ()  [unwired: 9 in, 2 out]
          }
        }
        n636 = local write "CAMERA ROI MAX TEMP"(TRUE ("CAMERA ROI MIN TEMP")) -> ()
      }
      frame "Advance" {
        n637 = local read "LIVE FEED MIN TEMP"() -> (w963:bool)
        n638 = local write "LIVE FEED MAX TEMP"(TRUE ("LIVE FEED MAX TEMP")) -> ()
        n639 = local read "CAMERA ROI MIN TEMP"() -> (w961:bool)
        n640 = case shown="True" w963 {
          selector: w963 -> [_ w970]
          frame False {
          }
          frame True {
            n641 = Not(x=w970) -> (.not. x?=w969:bool)
            n642 = local write "LIVE FEED MIN TEMP"(w969) -> ()
            n643 = call "CAMERA LIVE FEED FGV.vi"("Enum - Menu"=CAMERA_LIVE_FEED_ENUM."CAMERA MINIMIZE") -> ()  [unwired: 9 in, 2 out]
          }
        }
        n644 = local write "CAMERA ROI MAX TEMP"(TRUE ("CAMERA ROI MAX TEMP")) -> ()
        n645 = case shown="True" w961 {
          selector: w961 -> [_ w967]
          frame False {
          }
          frame True {
            n646 = Not(x=w967) -> (.not. x?=w966:bool)
            n647 = local write "CAMERA ROI MIN TEMP"(w966) -> ()
            n648 = call "IMAGE ANALYSIS.vi"("Enum"=POST_ANALYSIS_ENUM."MINIMIZE UI") -> ()  [unwired: 9 in, 2 out]
          }
        }
      }
      frame "Mooha" {
        n649 = local read "LIVE FEED MIN TEMP"() -> (w973:bool)
        n650 = local write "LIVE FEED MAX TEMP"(TRUE ("LIVE FEED MAX TEMP")) -> ()
        n651 = local read "CAMERA ROI MIN TEMP"() -> (w971:bool)
        n652 = case shown="True" w973 {
          selector: w973 -> [_ w980]
          frame False {
          }
          frame True {
            n653 = Not(x=w980) -> (.not. x?=w979:bool)
            n654 = local write "LIVE FEED MIN TEMP"(w979) -> ()
            n655 = call "CAMERA LIVE FEED FGV.vi"("Enum - Menu"=CAMERA_LIVE_FEED_ENUM."CAMERA MINIMIZE") -> ()  [unwired: 9 in, 2 out]
          }
        }
        n656 = local write "CAMERA ROI MAX TEMP"(TRUE ("CAMERA ROI MAX TEMP")) -> ()
        n657 = case shown="True" w971 {
          selector: w971 -> [_ w977]
          frame False {
          }
          frame True {
            n658 = Not(x=w977) -> (.not. x?=w976:bool)
            n659 = local write "CAMERA ROI MIN TEMP"(w976) -> ()
            n660 = call "IMAGE ANALYSIS.vi"("Enum"=POST_ANALYSIS_ENUM."MINIMIZE UI") -> ()  [unwired: 9 in, 2 out]
          }
        }
      }
    }
    n661 = local read "Auto Start Test"() -> (w784:bool)
    n662 = case shown="True" "sign in temp" {
      frame False {
      }
      frame True {
        w821 = 1 ("y")
        n663 = local read "USERNAME"() -> (w827:string)
        n664 = local read "USER ID"() -> (w824:string)
        n665 = call <vilib>:"Trim Whitespace.vi"("string"=w827) -> ("trimmed string"=w826:string)  [unwired: 1 in]
        n666 = call <vilib>:"Trim Whitespace.vi"("string"=w824) -> ("trimmed string"=w825:string)  [unwired: 1 in]
        n667 = String Length(string=w826) -> (length=w823:i32)
        n668 = String Length(string=w825) -> (length=w822:i32)
        n669 = Greater?(x=w823, y=w821) -> (0:w820:bool)
        n670 = Greater?(x=w822, y=w821) -> (0:w819:bool)
        n671 = And(x=w820, y=w819) -> (x .and. y?=w818:bool)
        n672 = case shown="True" w818 {
          frame False {
            n673 = property on="Sign In" class="Bool (strict)"("DisabledEnum"=T15."Disabled" ("Disabled")) -> ()  [unwired: 2 in, 2 out]
          }
          frame True {
            n674 = property on="Sign In" class="Bool (strict)"("DisabledEnum"=T15."Enabled" ("Disabled")) -> ()  [unwired: 2 in, 2 out]
          }
        }
      }
    }
    n675 = local read "Air Temperature"() -> (w801:bool)
    n676 = local read "Coefficient Of Friction"() -> (w802:bool)
    n677 = case shown="False" w784 {
      frame False {
        n678 = local read "Auto stop temp"() -> (w815:bool)
        n679 = case shown="True" w815 {
          frame False {
          }
          frame True {
            n680 = local write "Auto Start Temp"(TRUE ("Auto Start Temp")) -> ()
          }
        }
      }
      frame True {
        "Auto stop temp" <- TRUE ("Auto stop temp")
      }
    }
    n681 = local read "Humidity"() -> (w800:bool)
    n682 = case shown="\"HOME\"" w812 {
      frame "HOME" {
        n683 = local write "main tab sub"(enum32{"Page 1", "Page 2"}."Page 1" ("main tab sub")) -> ()
      }
      frame Default {
        n684 = local write "main tab sub"(enum32{"Page 1", "Page 2"}."Page 2" ("main tab sub")) -> ()
      }
    }
    n685 = case shown="True" w811 {
      selector: w811 -> [_ w1069]
      frame False {
      }
      frame True {
        n686 = Not(x=w1069) -> (.not. x?=w1068:bool)
        n687 = local write "Sign In"(w1068) -> ()
        n688 = local write "Main Dashboard Buttons"(T2."Test Setup" ("Main Dashboard Buttons")) -> ()
      }
    }
    n689 = case shown="\"Numeric Display\", Default" "Num/Graph" {
      frame "Numeric Display", Default {
        n690 = property on="Single/Multiple" class="RadioBtnsControl (strict)"("Visible"=FALSE) -> ()  [unwired: 2 in, 2 out]
        n691 = property on="Single - Graph" class="Ring (strict)"("Visible"=FALSE) -> ()  [unwired: 2 in, 2 out]
        n692 = local write "Main Tab Display"(T5."Dashboard 1" ("Main Tab Display")) -> ()
      }
      frame "Graph Display" {
        n693 = property on="Single/Multiple" class="RadioBtnsControl (strict)"("Visible"=TRUE) -> ()  [unwired: 2 in, 2 out]
        n694 = case shown="\"Multiple\"" "Single/Multiple" {
          frame "Single ", Default {
            n695 = property on="Single - Graph" class="Ring (strict)"("Visible"=TRUE) -> ()  [unwired: 2 in, 2 out]
            n696 = local write "Main Tab Display"(T5."Dashboard 3" ("Main Tab Display")) -> ()
          }
          frame "Multiple" {
            n697 = property on="Single - Graph" class="Ring (strict)"("Visible"=FALSE) -> ()  [unwired: 2 in, 2 out]
            n698 = local write "Main Tab Display"(T5."Dashboard 2" ("Main Tab Display")) -> ()
          }
        }
      }
    }
    n699 = local read "Stroke"() -> (w799:bool)
    n700 = local read "USERNAME"() -> (w805:string)
    n701 = local read "USER ID"() -> (w804:string)
    n702 = case shown="True" w802 {
      selector: w802 -> [_ w1020]
      frame False {
      }
      frame True {
        n703 = Not(x=w1020) -> (.not. x?=w1019:bool)
        n704 = local write "Coefficient Of Friction"(w1019) -> ()
        n705 = local write "Tab Control 2"(T7."Coefficient Of Friction" ("Tab Control 2")) -> ()
      }
    }
    n706 = case shown="True" w801 {
      selector: w801 -> [_ w1017]
      frame False {
      }
      frame True {
        n707 = Not(x=w1017) -> (.not. x?=w1015:bool)
        n708 = local write "Air Temperature"(w1015) -> ()
        n709 = local write "Tab Control 2"(T7."Air Temperature" ("Tab Control 2")) -> ()
      }
    }
    n710 = local write "Operator ID"(w804) -> ()
    n711 = case shown="True" w799 {
      selector: w799 -> [_ w1011]
      frame False {
      }
      frame True {
        n712 = Not(x=w1011) -> (.not. x?=w1009:bool)
        n713 = local write "Stroke"(w1009) -> ()
        n714 = local write "Tab Control 2"(T7."Stroke" ("Tab Control 2")) -> ()
      }
    }
    n715 = local write "tested by"(w805) -> ()
    n716 = case shown="True" w800 {
      selector: w800 -> [_ w1014]
      frame False {
      }
      frame True {
        n717 = Not(x=w1014) -> (.not. x?=w1012:bool)
        n718 = local write "Humidity"(w1012) -> ()
        n719 = local write "Tab Control 2"(T7."Humidity" ("Tab Control 2")) -> ()
      }
    }
    n720 = case shown="\"Analysis\"" "Main Dashboard Buttons" {
      tunnel: [T3."HOME" ("Main Tab") T3."Test Setup" ("Main Tab") T3."Acquire" ("Main Tab") T3."Adv Scar" ("Main Tab") T3."Adv Scar Report" ("Main Tab") T3."Compare Files" ("Main Tab") T3."About" ("Main Tab")] -> w809
      frame "Home", Default {
      }
      frame "Test Setup" {
      }
      frame "Dashboard" {
      }
      frame "Imaging" {
      }
      frame "Report" {
      }
      frame "Analysis" {
      }
      frame "About" {
      }
    }
    n721 = Wait (ms)(milliseconds to wait=u32 100) -> ()  [unwired: 1 out]
    n722 = local read "Main Tab Display"() -> (w803:T5)
    n723 = local write "Main Tab"(w809) -> ()
    n724 = case shown="\"Dashboard 3\"" w803 {
      frame "Dashboard 1", Default {
        n725 = property on="Reset Graph" class="Bool (strict)"("Visible"=FALSE) -> ()  [unwired: 2 in, 2 out]
      }
      frame "Dashboard 2" {
        n726 = property on="Reset Graph" class="Bool (strict)"("Visible"=TRUE) -> ()  [unwired: 2 in, 2 out]
      }
      frame "Dashboard 3" {
        n727 = property on="Reset Graph" class="Bool (strict)"("Visible"=TRUE) -> ()  [unwired: 2 in, 2 out]
      }
    }
    n728 = local read "SCAR MEASURMENT"() -> (w791:enum32{"Auto Scar", "Manual Scar"})
    n729 = local read "Humidity"() -> (w806:bool)
    n730 = local read "Cap Live Image"() -> (w788:bool)
    n731 = local read "Sample Temperature"() -> (w798:bool)
    n732 = local read "Air Temp vs Humidity"() -> (w796:bool)
    n733 = local read "Frequency"() -> (w797:bool)
    n734 = Equal?(x=w791, y=enum32{"Auto Scar", "Manual Scar"}."Auto Scar" ("SCAR MEASURMENT")) -> (x = y?=w787:bool)
    n735 = case shown="True" w806 {
      frame False {
        n736 = local write "Humidity On Command"(TRUE ("Humidity On Command")) -> ()
        n737 = case shown="True" "Humidity Off Command" {
          selector: "Humidity Off Command" -> [_ w1033]
          frame False {
          }
          frame True {
            n738 = Not(x=w1033) -> (.not. x?=w1032:bool)
            n739 = local write "Humidity Off Command"(w1032) -> ()
            n740 = local read "WriteHumidity"() -> (w1030:string[])
            n741 = local read "EVENT LOG"() -> (w1027:string)
            n742 = call "Event Log.vi"("Content"="Humidity Control Off" ("string"), "EVENT LOG"=w1027) -> ("EVENT LOG"=w1028:string)  [unwired: 8 in, 1 out]
            n743 = Insert Into Array(array=w1030, new element="R;1" ("new element/subarray")) -> (w1031:string[])  [unwired: 1 in]
            n744 = local write "EVENT LOG"(w1028) -> ()
            n745 = local write "WriteHumidity"(w1031) -> ()
          }
        }
      }
      frame True {
        n746 = case shown="True" "Humidity On Command" {
          selector: "Humidity On Command" -> [_ w1046]
          frame False {
          }
          frame True {
            n747 = local read "Set Rh"() -> (w1041:dbl)
            n748 = Not(x=w1046) -> (.not. x?=w1045:bool)
            n749 = local write "Humidity On Command"(w1045) -> ()
            n750 = Number To Fractional String(number=w1041, precision (6)=i16 2) -> (F-format string=w1038:string)  [unwired: 2 in]
            n751 = local read "WriteHumidity"() -> (w1043:string[])
            n752 = Concatenate Strings("M;" ("new element/subarray"), w1038) -> (w1042:string)
            n753 = Concatenate Strings("Humidity Set to : " ("string"), w1038, "% RH" ("string")) -> (w1036:string)
            n754 = Insert Into Array(array=w1043, new element=w1042) -> (w1044:string[])  [unwired: 1 in]
            n755 = disable-structure shown="Enabled" {
              disable-tunnel: w1036 -> [_ _]
              frame Enabled {
                n756 = local read "EVENT LOG"() -> (w1049:string)
                n757 = call "Event Log.vi"("Content"="Humidity Control On", "EVENT LOG"=w1049) -> ("EVENT LOG"=w1050:string)  [unwired: 8 in, 1 out]
                n758 = local write "EVENT LOG"(w1050) -> ()
              }
              frame Disabled {
              }
            }
            n759 = local write "WriteHumidity"(w1044) -> ()
          }
        }
        n760 = local write "Humidity Off Command"(TRUE ("Humidity Off Command")) -> ()
      }
    }
    n761 = local read "TEST STANDARD"() -> (w794:T4)
    n762 = And(x=w788, y=w787) -> (x .and. y?=w789:bool)
    n763 = case shown="True" w789 {
      selector: w789 -> [_ w839]
      tunnel: errorcluster {"status"=FALSE, "code"=0, "source"=""} ("error in (no error) 3") -> [_ w840]
      frame False {
      }
      frame True {
        n764 = stacked-sequence {
          tunnel: w840 -> [_ _ _ _ _ _ _ w884]
          tunnel: w839 -> [_ _ _ _ _ w867 _ _]
          frame #0 {
            n765 = call "CAMERA LIVE FEED FGV.vi"("Enum - Menu"=CAMERA_LIVE_FEED_ENUM."CAMERA MINIMIZE") -> ()  [unwired: 9 in, 2 out]
          }
          frame #1 {
            n766 = property on="Auto Scar Check  2" class="Clust (strict)"("Visible"=TRUE) -> ()  [unwired: 2 in, 2 out]
          }
          frame #2 {
            n767 = String To Path(string="C:\\LAB-IQ\\Image Calibrate v01.dcf") -> (path=w845:path)
            n768 = Open/Create/Replace File ("Open File")(file path (use dialog)=w845) -> (refnum out=w846:refnum<file>)  [unwired: 5 in, 2 out]
            n769 = for {
              N: 4 -> [_]
              tunnel: w846 -> [w852]
              i -> [w848]
              n770 = Read from Text File ("Read File")(file (use dialog)=w852) -> (text=w853:string)  [unwired: 3 in, 3 out]
              n771 = String Subset(string=w853, offset (0)=6, length (rest)=10 ("length (rest)")) -> (substring=w849:string)
              n772 = Fract/Exp String To Number(string=w849) -> (number=w847:dbl)  [unwired: 3 in, 1 out]
              n773 = case shown="0" w848 {
                tunnel: w847 -> [w854 w855 _ w856 _]
                frame 0 {
                  "5x Gain" <- w854
                }
                frame 1 {
                  "10x Gain" <- w855
                }
                frame 2 {
                }
                frame 3 {
                  "100x gain" <- w856
                }
                frame 4, Default {
                }
              }
            }
          }
          frame #3 {
            n774 = local read "FILE 3"() -> (w862:string)
            n775 = call <vilib>:"Trim Whitespace.vi"("string"="C:\\LAB-IQ\\images\\") -> ("trimmed string"=w864:string)  [unwired: 1 in]
            n776 = String To Path(string=w864) -> (path=w863:path)
            n777 = Concatenate Strings(w862, ".png" ("string")) -> (w861:string)
            n778 = Build Path(base path=w863, name or relative path=w861) -> (appended path=w859:path)
            "Image path" <- w859
            n779 = Path To String(path=w859) -> (string=w858:string)
            n780 = call "CAMERA LIVE FEED FGV.vi"("Enum - Menu"=CAMERA_LIVE_FEED_ENUM."CAMERA SAVE", "Image Path"=w858) -> ()  [unwired: 8 in, 2 out]
          }
          frame #4 {
            n781 = One Button Dialog(message="Image saved successfully") -> ()  [unwired: 1 in, 1 out]
          }
          frame #5 {
            n782 = local read "Magnification len live scar"() -> (w878:string)
            n783 = Not(x=w867) -> (.not. x?=w868:bool)
            n784 = local write "Cap Live Image"(w868) -> ()
            n785 = case shown="\"5x\", Default" w878 {
              tunnel: [w879 w880] -> w877
              frame "5x", Default {
                n786 = local read "5x Gain"() -> (w879:dbl)
              }
              frame "10x" {
                # "5x"
                n787 = local read "10x Gain"() -> (w880:dbl)
              }
            }
            n788 = local read "Image path"() -> (w876:path)
            n789 = local read "FILE 3"() -> (w869:string)
